vi "Global_SEN_Data Out.vi"() -> ()   [LabVIEW 2020, in "PigeonIMU_SEN_ts.lvlib"]
uses:
  PigeonIMU_SEN_ts.lvlib
  Shared Code/TypeDefs/Cluster_Unity Yaw-Pitch-Roll.ctl
  Shared Code/TypeDefs/Dial_Compase heading unit circle CCW positive.ctl
panel:
  out "Sen_Pigeon_Swinging":bool
  out "Sen_Pigeon_Running":bool
  out "Sen_Pigeon_YawPitchRoll":T1 {"Roll" scale format="%.3f"; "Pitch" scale format="%.3f"; "Yaw" scale format="%.3f"}
  # "The Names of the Data items in the Global Variable MUST describe who the Single Writer is\nFor Sensor Globals the the naming convention is\n   \nSEN_Lib Name_Data Name\n\nExamples:\nSEN_Gyro_Angle\nSEN_Sonar_Distance"
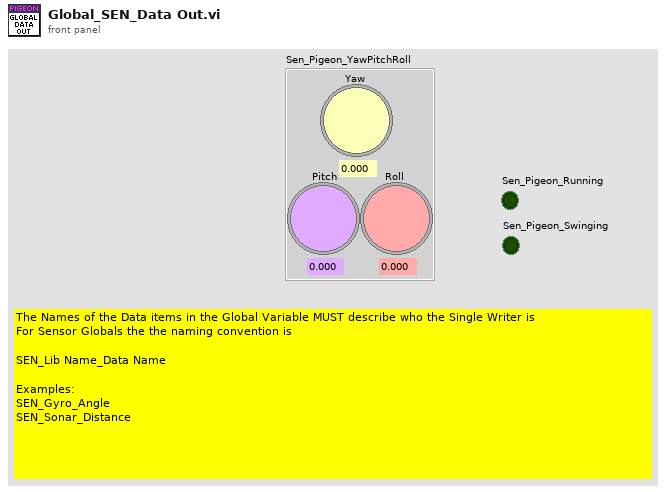
[diagram p1: front panel]
types:
  T1 = typedef "Cluster_Unity Yaw-Pitch-Roll.ctl" = cluster{"Yaw":T2, "Pitch":T2, "Roll":T2}
  T2 = typedef "Dial_Compase heading unit circle CCW positive.ctl" = dbl
diagram:
